vi "KE622x -- Arm Init Sweep.vi"(0 "Resource In":refnum<visa-resource-name>, 1 "Check For SCPI Errors? (T)":bool=TRUE, 2 "Init Sweep? (T)":bool=TRUE, 7 "Sweep Type":T1, 11 "error in (no error)":errorcluster) -> (4 "Resource Out (dupl)":refnum<visa-resource-name>, 15 "error out":errorcluster)   [LabVIEW 2010, in "Keithley 622x.lvlib"]
doc: "Used to arm a given sweep type (Linear, Log, or List sweep), and also optionally start the sweep."
uses:
  Keithley 622x.lvlib
  <instrlib>/Keithley 622x LV 2009/Configure/Source/Typedefs/KE622x -- Sweep Type.ctl
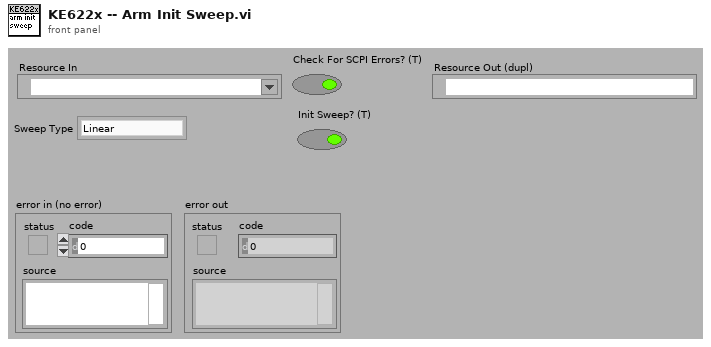
[diagram p1: front panel]
types:
  T1 = typedef "Keithley 622x.lvlib/KE622x -- Sweep Type.ctl" = enum16{"Linear", "Log", "List"}
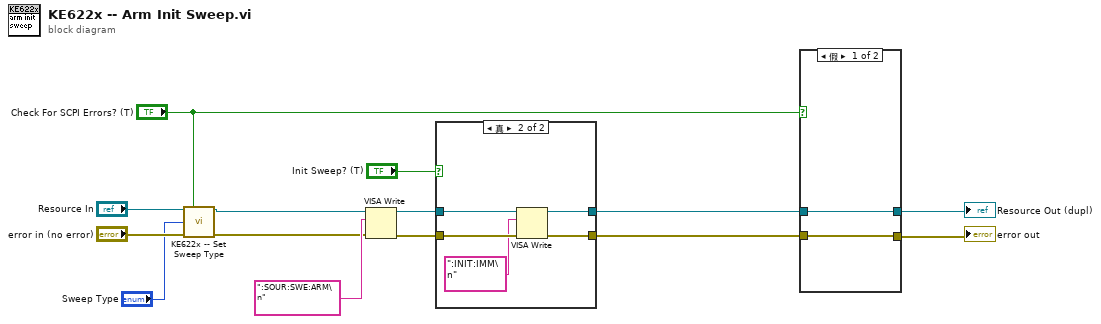
[diagram p0: block diagram]
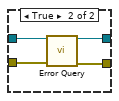
[diagram p3: hidden frame]
diagram:
  n1 = call "KE622x -- Set Sweep Type.vi"("Resource In"="Resource In", "Check For SCPI Errors? (T)"="Check For SCPI Errors? (T)", "Sweep Type"="Sweep Type", "error in (no error)"="error in (no error)") -> ("Resource Out (dupl)"=w2:refnum<visa-resource-name>, "error out"=w3:errorcluster)  [unwired: 10 in]
  n2 = VISA Write(VISA resource name=w2, write buffer=":SOUR:SWE:ARM\n" ("format string"), error in (no error)=w3) -> (VISA resource name out=w10:refnum<visa-resource-name>, error out=w9:errorcluster)  [unwired: 1 out]
  n3 = case shown="真" "Init Sweep? (T)" {
    tunnel: w10 -> [w16 w21]
    tunnel: w9 -> [w15 w20]
    tunnel: [w15 w18] -> w8
    tunnel: [w16 w17] -> w7
    frame False {
    }
    frame True {
      n4 = VISA Write(VISA resource name=w21, write buffer=":INIT:IMM\n", error in (no error)=w20) -> (VISA resource name out=w17:refnum<visa-resource-name>, error out=w18:errorcluster)  [unwired: 1 out]
    }
  }
  n5 = case shown="假" "Check For SCPI Errors? (T)" {
    tunnel: w7 -> [w23 w27]
    tunnel: w8 -> [w22 w26]
    tunnel: [w22 w25] -> w13
    tunnel: [w23 w24] -> w14
    frame False {
    }
    frame True {
      n6 = call "Error Query.vi"("VISA Resource In"=w27, "error in (no error)"=w26) -> ("VISA Resource Out (dupl)"=w24:refnum<visa-resource-name>, "error out"=w25:errorcluster)  [unwired: 10 in, 2 out]
    }
  }
  "Resource Out (dupl)" <- w14
  "error out" <- w13
